vi "CoreState_Init.vi"(8 "error in (no error)":errorcluster, 11 "MB Slave Simulator Base in":refnum<class "MB Slave Simulator Base.lvclass">) -> (0 "error out":errorcluster, 3 "MB Slave Simulator Base out":refnum<class "MB Slave Simulator Base.lvclass">)   [LabVIEW 2021, in "MB Slave Simulator Base.lvclass"]
uses:
  MB Slave Simulator Base.lvclass
  TypeDefs/dvr_type.ctl
  TypeDefs/_PARMS.ctl
  <userlib>/S2 Labs/Module Framework/Modules/Base/Launch Module Typdef.ctl
  <userlib>/S2 Labs/Module Framework/Modules/Base/Launch Module Parms.ctl
  TypeDefs/state_vars.ctl
  MB Slave Simulator Base.lvclass/MB Slave Simulator Base.ctl
  <userlib>/S2 Labs/Module Framework/Modules/Modbus/Modbus Slave Base/Modbus Slave Base.lvclass
  <userlib>/S2 Labs/Module Framework/Modules/Base/Module.lvclass
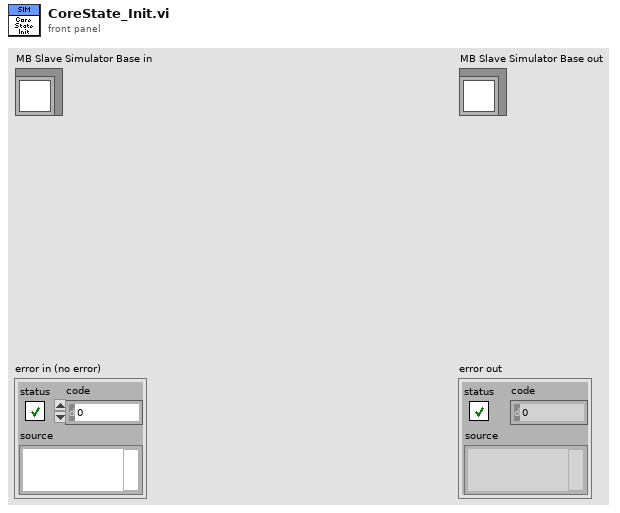
[diagram p1: front panel]
types:
  T1 = typedef "MB Slave Simulator Base.lvclass/dvr_type.ctl" = cluster{"_PARMS":T2, "state_vars":T5}
  T2 = typedef "MB Slave Simulator Base.lvclass/_PARMS.ctl" = cluster{"ch_alias":string[], "ch_units":string[], "Modules to Launch":T3[]}
  T3 = typedef "Module.lvclass/Launch Module Typdef.ctl" = cluster{"Module":string, "Parameters":T4}
  T4 = typedef "Module.lvclass/Launch Module Parms.ctl" = cluster{"Name":string, "Arguments":string[], "Show FP?":bool}
  T5 = typedef "MB Slave Simulator Base.lvclass/state_vars.ctl" = cluster{"Initialized":bool}
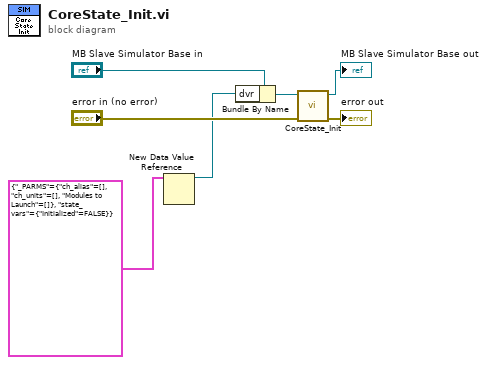
[diagram p0: block diagram]
diagram:
  n1 = New Data Value Reference(data value=T1 {"_PARMS"={"ch_alias"=[], "ch_units"=[], "Modules to Launch"=[]}, "state_vars"={"Initialized"=FALSE}} ("dvr_type")) -> (data value reference=w1:refnum<data-value>)  [unwired: 1 in, 1 out]
  n2 = Bundle By Name(cluster="MB Slave Simulator Base in", "dvr"=w1) -> (w2:refnum<class "MB Slave Simulator Base.lvclass">)
  n3 = call-parent "CoreState_Init.vi"("error in (no error)"="error in (no error)", "Modbus Slave Base in"=w2) -> ("error out"=→"error out":errorcluster, "Modbus Slave Base out"=→"MB Slave Simulator Base out":refnum<class "MB Slave Simulator Base.lvclass">)  [unwired: 8 in]
